vi "command.vi"(7 "LabVIEW Web Service Request":refnum<class "Web Request.lvclass">) -> ()   [LabVIEW 2017]
uses:
  <vilib>/wsapi/Web Request.lvclass
  states.ctl
panel:
  # "Use the Web Service Request input terminal to call the VIs on the Web Services palette. Do not remove it from the connector pane unless you don't need access to the palette."
  # "Each additional control wired to the connector pane will be available as an input in the URL. To include an indicator in terminal-mode output (the default setting), it must also be wired to the connector pane."
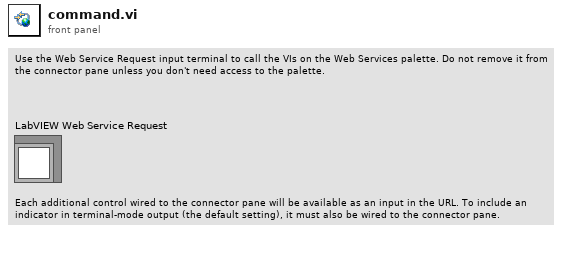
[diagram p1: front panel]
types:
  T1 = typedef "states.ctl" = enum16{"waiting for command", "go to ground floor", "go to floor 1", "go to floor 2", "drop cart"}
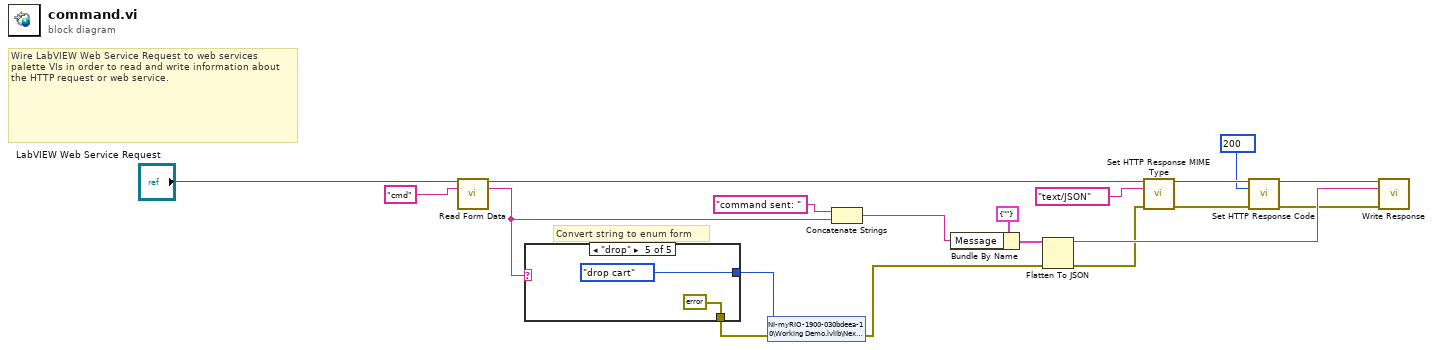
[diagram p0: block diagram]
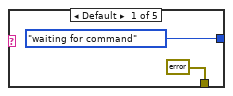
[diagram p2: hidden frame]
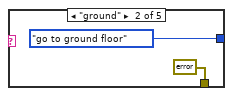
[diagram p3: hidden frame]
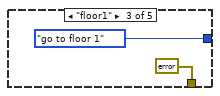
[diagram p4: hidden frame]
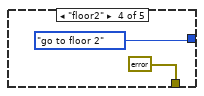
[diagram p5: hidden frame]
diagram:
  w1 = 200 items=["100"=100, "101"=101, "200"=200, "201"=201, "202"=202, "203"=203, "204"=204, "205"=205, "206"=206, "300"=300, "301"=301, "302"=302, "303"=303, "304"=304, "305"=305, "306"=306, "307"=307, "400"=400, "401"=401, "402"=402, "403"=403, "404"=404, "405"=405, "406"=406, "407"=407, "408"=408, "409"=409, "410"=410, "411"=411, "412"=412, "413"=413, "414"=414, "415"=415, "416"=416, "417"=417, "500"=500, "501"=501, "502"=502, "503"=503, "504"=504, "505"=505] ("response code (200)")
  # "Convert string to enum form"
  # "Wire LabVIEW Web Service Request to web services palette VIs in order to read and write information about the HTTP request or web service."
  n1 = call <vilib>:"Read Form Data.vi"("LabVIEW Web Service Request"="LabVIEW Web Service Request", "key"="cmd") -> ("LabVIEW Web Service Request out"=w11:refnum<class "Web Request.lvclass">, "value"=w5:string)  [unwired: 10 in, 2 out]
  n2 = case shown="\"drop\"" w5 {
    tunnel: [states."waiting for command" ("states") states."go to ground floor" ("states") states."go to floor 1" ("states") states."go to floor 2" ("states") states."drop cart" ("states")] -> w12
    tunnel: [errorcluster {"status"=FALSE, "code"=0, "source"=""} ("error in (no error)") errorcluster {"status"=FALSE, "code"=0, "source"=""} ("error in (no error)") errorcluster {"status"=FALSE, "code"=0, "source"=""} ("error in (no error)") errorcluster {"status"=FALSE, "code"=0, "source"=""} ("error in (no error)") errorcluster {"status"=FALSE, "code"=0, "source"=""} ("error in (no error)")] -> w6
    frame Default {
    }
    frame "ground" {
    }
    frame "floor1" {
    }
    frame "floor2" {
    }
    frame "drop" {
    }
  }
  n3 = shared-variable "NI-myRIO-1900-030bdeea-10\\Working Demo.lvlib\\Next State"(w12, error in=w6) -> (error out=w7:errorcluster)
  n4 = Concatenate Strings("command sent: ", w5) -> (w4:string)
  n5 = Bundle By Name(cluster=cluster{"Message":string} {"Message"=""} ("input cluster"), "Message"=w4) -> (w9:cluster{"Message":string})
  n6 = Flatten To JSON(anything=w9, error in (no error)=w7) -> (JSON string=w19:string, 11:w14:errorcluster)  [unwired: 1 in]
  n7 = call <vilib>:"Set HTTP Response MIME Type.vi"("LabVIEW Web Service Request"=w11, "MIME type (text/html)"="text/JSON", "error in (no error)"=w14) -> ("LabVIEW Web Service Request out"=w3:refnum<class "Web Request.lvclass">, "error out"=w2:errorcluster)  [unwired: 11 in]
  n8 = call <vilib>:"Set HTTP Response Code.vi"("LabVIEW Web Service Request"=w3, "response code (200)"=w1, "error in (no error)"=w2) -> ("LabVIEW Web Service Request out"=w16:refnum<class "Web Request.lvclass">, "error out"=w17:errorcluster)  [unwired: 11 in]
  n9 = call <vilib>:"Write Response.vi"("LabVIEW Web Service Request"=w16, "response string"=w19, "error in (no error)"=w17) -> ()  [unwired: 11 in, 2 out]
